vi "MultipleTests.vi"() -> ()   [LabVIEW 2018]
uses:
  FGV/FGV_mods.ctl
  <vilib>/Heliosphere Research LLC/Advanced Plotting Toolkit/api_core/NewPlotType.ctl
  <vilib>/Analysis/1siggen.llb/Ramp Pattern by Samples.vi
  <vilib>/Analysis/NI_AALBase.lvlib
  <vilib>/Heliosphere Research LLC/Advanced Plotting Toolkit/Advanced Plotting Toolkit.lvlib
panel:
  out "Pasta atual":string
  in  "dir_pics":path caption="Directory pictures"
  out "Progresso":dbl(slide) scale=0.0..100.0
  in  "Channels per graph":i32=1
  out "error out":errorcluster
  out "Polar":picture
  in  "file":path caption="Directory tests"
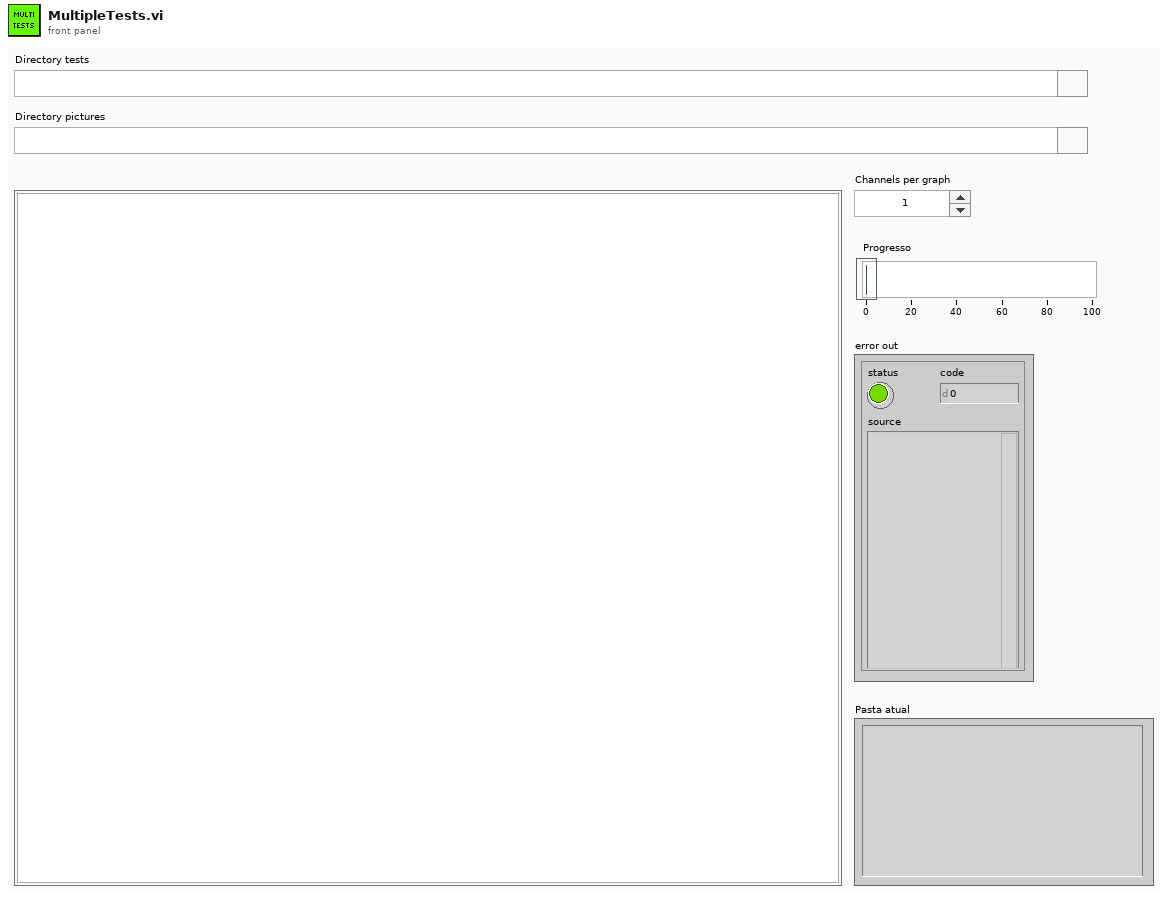
[diagram p1: front panel]
types:
  T1 = typedef "FGV_mods.ctl" = enum16{"Init", "get_config", "get_hits", "set_file", "open_file", "get_startTime", "close"}
  T2 = typedef "Advanced Plotting Toolkit.lvlib/NewPlotType.ctl" = enum16{"Rectangular Axes", "Polar Axes"}
  T3 = typedef "hit_data.ctl" = cluster{"channel":u8, "time":dbl, "parameters":cluster{"riseTime":u32, "countsToPeak":u32, "counts":u32, "energy":u32, "duration":u32, "amplitude":u32, "RMS":u32, "ASL":u32, "gain":u32, "THR":u32, "preAmp":u32, "avrFreq":u32}}
  T4 = typedef "polar_data.ctl" = cluster{"t0":dbl, "conts":dbl[], "amps":dbl[]}
  T5 = typedef "Advanced Plotting Toolkit.lvlib/PlotID.ctl" = i32
  T6 = typedef "imagedata.ctl" = cluster{"image type":i32, "image depth":i32, "image":u8[], "mask":u8[], "colors":u32[], "Rectangle":cluster{"left":i16, "top":i16, "right":i16, "bottom":i16}}
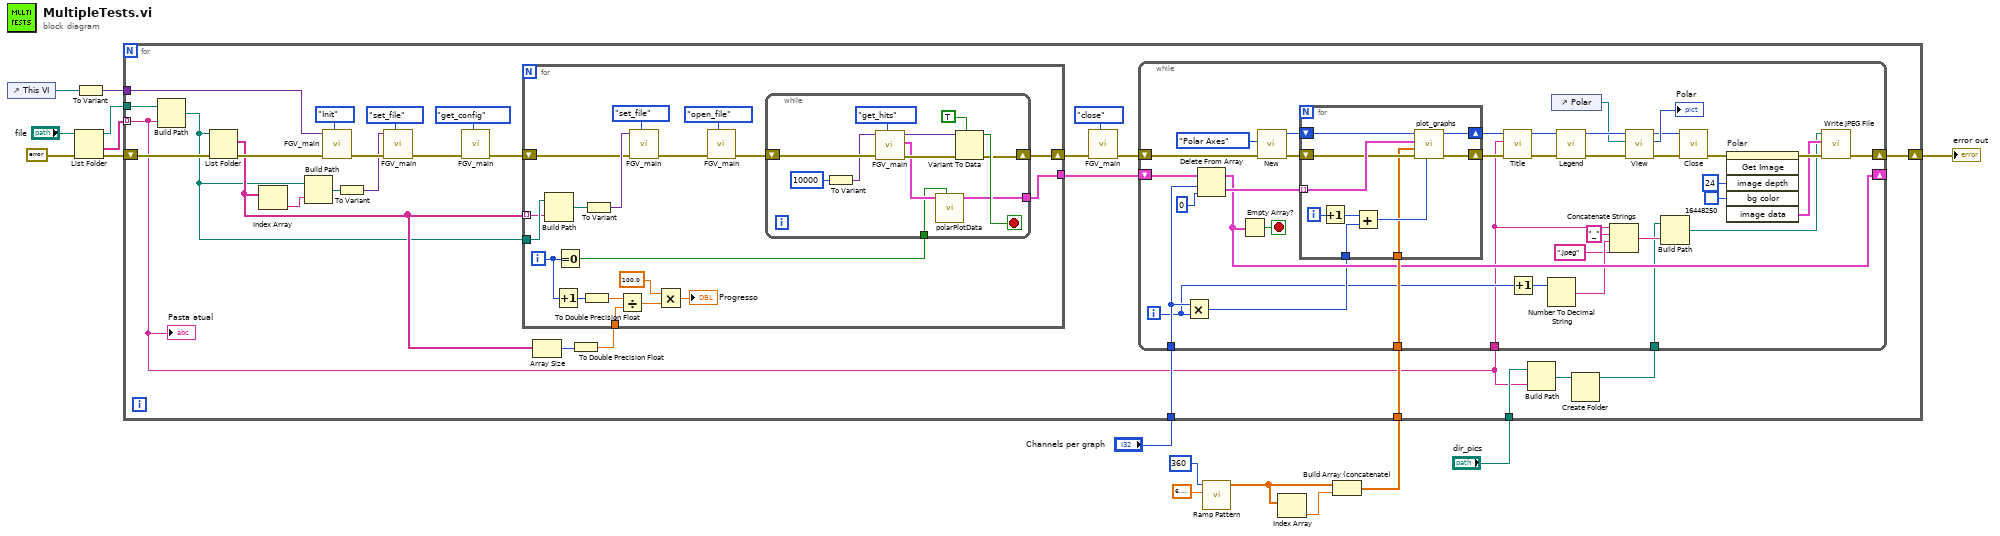
[diagram p0: block diagram]
diagram:
  n1 = control-ref of="This VI"() -> (w15:refnum<vi>)
  n2 = List Folder(path="file", error in=errorcluster {"status"=FALSE, "code"=0, "source"=""} ("Error Out")) -> (path out=w4:path, folder names=w1:string[], error out=w3:errorcluster)  [unwired: 2 in, 1 out]
  n3 = To Variant(anything=w15) -> (Variant=w14:variant)
  n4 = call-poly <vilib>:"Ramp Pattern.vi"("end"=6.283185307179586, "samples"=360) -> ("Ramp Pattern"=w6:dbl[])  [unwired: 8 in, 1 out]
  n5 = Index Array(array=w6) -> (element=w11:dbl)  [unwired: 1 in]
  n6 = Build Array (concatenate)(w6, w11) -> (w10:dbl[])
  n7 = for {
    tunnel: w14 -> [w38]
    tunnel: w4 -> [w21]
    tunnel: w10 -> [w28]
    tunnel: "Channels per graph" -> [w26]
    tunnel: "dir_pics" -> [w19]
    shift-right: [w27] -> w9
    shift-left: w3 -> [w22]
    tunnel: w1 -> [w18] mode=indexing
    n8 = Build Path(base path=w21, name or relative path=w18) -> (appended path=w20:path)
    n9 = List Folder(path=w20, error in=w22) -> (filenames=w32:string[], error out=w37:errorcluster)  [unwired: 2 in, 2 out]
    n10 = Index Array(array=w32) -> (element=w43:string)  [unwired: 1 in]
    n11 = Build Path(base path=w20, name or relative path=w43) -> (appended path=w42:path)
    n12 = call "FGV_main.vi"("FGV_mods"=FGV_mods."Init", "Error In"=w37, "DataIn"=w38) -> ("Error Out"=w41:errorcluster)  [unwired: 6 in, 2 out]
    n13 = To Variant(anything=w42) -> (Variant=w33:variant)
    n14 = call "FGV_main.vi"("FGV_mods"=FGV_mods."set_file", "Error In"=w41, "DataIn"=w33) -> ("Error Out"=w35:errorcluster)  [unwired: 6 in, 2 out]
    n15 = call "FGV_main.vi"("FGV_mods"=FGV_mods."get_config", "Error In"=w35) -> ("Error Out"=w34:errorcluster)  [unwired: 7 in, 2 out]
    n16 = Array Size(array=w32) -> (size(s)=w31:i32)
    n17 = To Double Precision Float(number=w31) -> (double precision float=w30:dbl)
    n18 = for {
      tunnel: [w60] -> w29
      shift-right: [w53] -> w24
      shift-left: w34 -> [w52]
      tunnel: w20 -> [w57]
      tunnel: w32 -> [w56] mode=indexing
      tunnel: w30 -> [w49]
      i -> [w45]
      n19 = Build Path(base path=w57, name or relative path=w56) -> (appended path=w55:path)
      n20 = Increment(x=w45) -> (x+1=w51:i32)
      n21 = Equal To 0?(x=w45) -> (x = 0?=w44:bool)
      n22 = To Double Precision Float(number=w51) -> (double precision float=w50:dbl)
      n23 = To Variant(anything=w55) -> (Variant=w54:variant)
      n24 = Divide(x=w50, y=w49) -> (x/y=w48:dbl)
      n25 = call "FGV_main.vi"("FGV_mods"=FGV_mods."set_file", "Error In"=w52, "DataIn"=w54) -> ("Error Out"=w58:errorcluster)  [unwired: 6 in, 2 out]
      n26 = Multiply(x=100.0, y=w48) -> (x*y=→"Progresso":dbl)
      n27 = call "FGV_main.vi"("FGV_mods"=FGV_mods."open_file", "Error In"=w58) -> ("Error Out"=w61:errorcluster)  [unwired: 7 in, 2 out]
      n28 = while {
        shift-right: [w67] -> w53
        shift-left: w61 -> [w73]
        tunnel: [w65] -> w60
        tunnel: w44 -> [w63]
        stop <- w68 stop-if-true
        n29 = To Variant(anything=10000) -> (Variant=w71:variant)
        n30 = call "FGV_main.vi"("FGV_mods"=FGV_mods."get_hits", "Error In"=w73, "DataIn"=w71) -> ("Error Out"=w66:errorcluster, "hits"=w64:T3[], "DataOut"=w70:variant)  [unwired: 6 in]
        n31 = call "polarPlotData.vi"("reset"=w63, "hits"=w64) -> ("polar_plot_data"=w65:T4[])  [unwired: 9 in]
        n32 = Variant To Data(error in=w66, type=TRUE, Variant=w70) -> (data=w68:bool, error out=w67:errorcluster)
      }
    }
    n33 = call "FGV_main.vi"("FGV_mods"=FGV_mods."close", "Error In"=w24) -> ("Error Out"=w23:errorcluster)  [unwired: 7 in, 2 out]
    n34 = Build Path(base path=w19, name or relative path=w18) -> (appended path=w17:path)
    n35 = Create Folder(path (use dialog)=w17) -> (created path=w16:path)  [unwired: 2 in, 2 out]
    n36 = while {
      tunnel: w28 -> [w102]
      shift-right: [w88] -> w27
      shift-left: w23 -> [w101]
      shift-right: [w97] -> _
      shift-left: w29 -> [w100]
      tunnel: w26 -> [w94]
      tunnel: w18 -> [w81]
      tunnel: w16 -> [w75]
      i -> [w83]
      stop <- w96 stop-if-true
      n37 = Multiply(x=w94, y=w83) -> (x*y=w95:i32)
      n38 = Delete From Array(array=w100, length=w94, index=0) -> (deleted portion=w98:T4[], array with subset deleted=w97:T4[])
      n39 = Empty Array?(array=w97) -> (empty?=w96:bool)
      n40 = call <vilib>:"New.vi"("error in (no error)"=w101, "Plot Type"=NewPlotType."Polar Axes") -> ("error out"=w108:errorcluster, "Plot ID"=w107:T5)  [unwired: 8 in]
      n41 = for {
        tunnel: w102 -> [w112]
        tunnel: w98 -> [w121] mode=indexing
        shift-right: [w118] -> w87
        shift-left: w108 -> [w120]
        shift-right: [w117] -> w84
        shift-left: w107 -> [w119]
        tunnel: w95 -> [w114]
        i -> [w116]
        n42 = Increment(x=w116) -> (x+1=w115:i32)
        n43 = Add(x=w115, y=w114) -> (x+y=w113:i32)
        n44 = call "plot_graphs.vi"("channel"=w113, "error in"=w120, "angs"=w112, "polar_data"=w121, "Plot ID"=w119) -> ("error out"=w118:errorcluster, "Plot ID out"=w117:T5)  [unwired: 5 in]
      }
      n45 = call <vilib>:"Title.vi"("error in (no error)"=w87, "Title"=w81, "Plot ID"=w84) -> ("error out"=w86:errorcluster, "Plot ID out"=w85:T5)  [unwired: 7 in]
      n46 = Increment(x=w83) -> (x+1=w82:i32)
      n47 = Number To Decimal String(number=w82) -> (decimal integer string=w80:string)  [unwired: 1 in]
      n48 = control-ref of="Polar"() -> (w106:refnum<vi>)
      n49 = call <vilib>:"Legend.vi"("error in (no error)"=w86, "Plot ID"=w85) -> ("error out"=w110:errorcluster, "Plot ID Out"=w111:T5)  [unwired: 8 in]
      n50 = Concatenate Strings(w81, "_" ("string"), w80, ".jpeg" ("string")) -> (w77:string)
      n51 = call <vilib>:"View.vi"("error in (no error)"=w110, "Ref for Sizing"=w106, "Plot ID"=w111) -> ("error out"=w104:errorcluster, "Picture"=→"Polar":picture, "Plot ID Out"=w103:T5)  [unwired: 6 in]
      n52 = Build Path(base path=w75, name or relative path=w77) -> (appended path=w76:path)
      n53 = call <vilib>:"Close.vi"("error in (no error)"=w104, "Plot ID"=w103) -> ("error out"=w93:errorcluster)  [unwired: 9 in]
      n54 = invoke on="Polar" class="Pict" method="Get Image"(error in=w93, "image depth"=24 ("Image Depth"), "bg color"=u32 16448250) -> (error out=w90:errorcluster, "image data"=w89:T6)  [unwired: 3 in, 4 out]
      n55 = call <vilib>:"Write JPEG File.vi"("error in (no error)"=w90, "image data"=w89, "path to JPEG file"=w76) -> ("error out"=w88:errorcluster)  [unwired: 7 in, 1 out]
    }
    "Pasta atual" <- w18
  }
  "error out" <- w9
